vi "Send speed logging start notifier in live protocols.vi"   [LabVIEW 2020]
uses:
  Typedefs/Speed acq notifier data.ctl
  Typedefs/Notifier Function.ctl
  Global Variables/General Globals.vi
types:
  T1 = typedef "Notifier Function.ctl" = enum16{"Send notifier", "Wait on notification", "Release notifier"}
  T2 = typedef "Speed acq notifier data.ctl" = cluster{"Log speed data":bool, "File path":path, "Initial timestamp":timestamp}
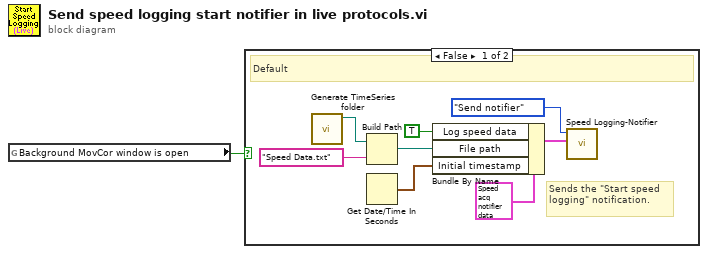
[diagram p0: block diagram]
diagram:
  n1 = global read "General Globals.vi" "Background MovCor window is open"() -> (w1:bool)
  n2 = case shown="False" w1 {
    frame False {
      # "Sends the \"Start speed logging\" notification."
      # "Default"
      n3 = call "Generate TimeSeries folder.vi"() -> ("Timelapse folder path"=w6:path)  [unwired: 10 in, 1 out]
      n4 = Build Path(base path=w6, name or relative path="Speed Data.txt") -> (appended path=w8:path)
      n5 = Get Date/Time In Seconds() -> (seconds since 1Jan1904=w2:timestamp)
      n6 = Bundle By Name(cluster=T2 {"Log speed data"=FALSE, "File path"=path "", "Initial timestamp"=timestamp(0 s since 1904-01-01)} ("Value to send"), "Log speed data"=TRUE ("Log?"), "File path"=w8, "Initial timestamp"=w2) -> (w5:T2)
      n7 = call "Speed Logging-Notifier.vi"("Value to send"=w5, "Notifier Function"=Notifier_Function."Send notifier") -> ()  [unwired: 7 in, 3 out]
    }
    frame True {
      # "Background movCor / Do not generate file"
    }
  }
